vi "Normalize Elements.vi"(8 "error in (no error)":errorcluster, 9 "Hierarchies":cluster{"Hierarchy":string[]}[](array[cluster]), 10 "Elements in":refnum<class "Config Element.lvclass">[](array[class])) -> (0 "error out":errorcluster, 2 "Elements":refnum<class "Config Element.lvclass">[](array[class]))   [LabVIEW 2020, in "CDM-Config.lvlib" / "Config Manager.lvclass"]
uses:
  Config Manager.lvclass
  Config Element/Config Element.lvclass
  <vilib>/Utility/miscctls.llb/LVMapReplaceAction.ctl
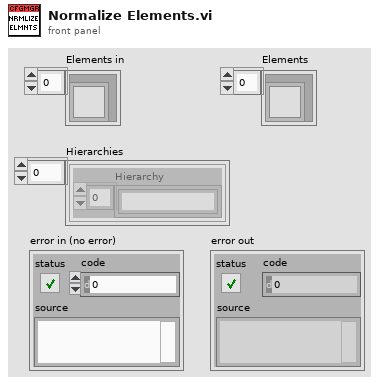
[diagram p1: front panel]
types:
  T1 = map{string[], refnum<class "Config Element.lvclass">}
  T2 = typedef "LVMapReplaceAction.ctl" = enum32{"Modify Entry only if found", "Add or Modify Entry", "Delete Entry"}
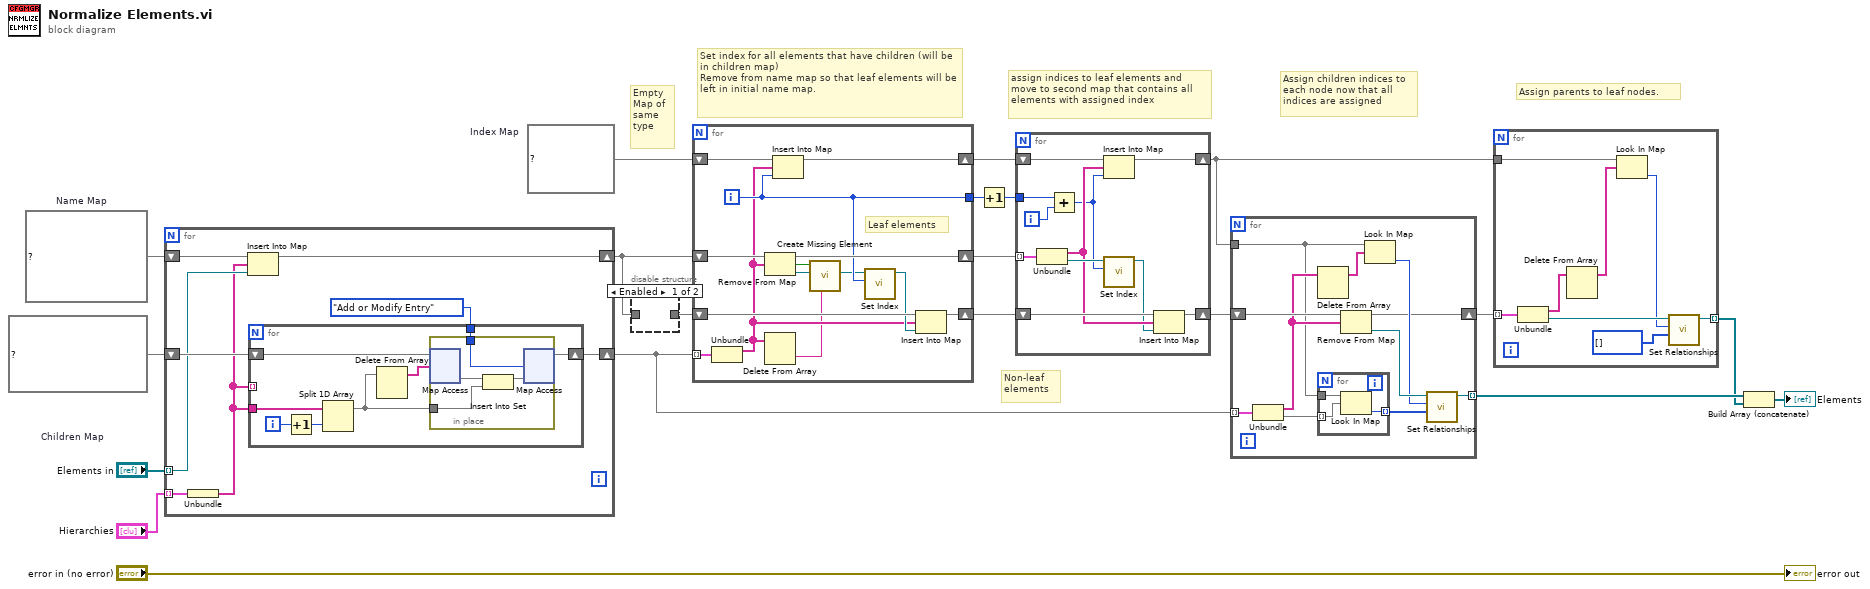
[diagram p0: block diagram]
diagram:
  w17 = map{string[], i32} {}  # Index Map
  w18 = T1 {}  # Name Map
  w19 = map{string[], set{string[]}} {}  # Children Map
  # "Assign parents to leaf nodes."
  # "Non-leaf elements"
  # "Assign children indices to each node now that all indices are assigned"
  # "assign indices to leaf elements and move to second map that contains all elements with assigned index"
  # "Set index for all elements that have children (will be in children map)\nRemove from name map so that leaf elements will be left in initial name map."
  # "Empty Map of same type"
  n1 = for {
    tunnel: "Elements in" -> [w24] mode=indexing
    shift-right: [w25] -> w11
    shift-left: w19 -> [w28]
    shift-right: [w26] -> w16
    shift-left: w18 -> [w27]
    tunnel: "Hierarchies" -> [w22] mode=indexing
    n2 = Unbundle(w22) -> ("Hierarchy"=w21:string[])
    n3 = Insert Into Map(map in=w27, key=w21, value=w24) -> (map out=w26:T1)  [unwired: 2 out]
    n4 = for {
      shift-right: [w35] -> w25
      shift-left: w28 -> [w36]
      tunnel: w21 -> [w32]
      tunnel: LVMapReplaceAction."Add or Modify Entry" ("action") -> [w29]
      tunnel: w21 -> [_] mode=indexing
      i -> [w34]
      n5 = Increment(x=w34) -> (x+1=w33:i32)
      n6 = Split 1D Array(array=w32, index=w33) -> (first subarray=w30:string[])  [unwired: 1 out]
      n7 = Delete From Array(array=w30) -> (array with subset deleted=w31:string[])  [unwired: 2 in, 1 out]
      n8 = in-place {
        in-place-border: w30 -> [w38]
        in-place-border: w29 -> [w37]
        n9 = in-place-map #1(w36, w31) -> (w40:set{string[]})  [unwired: 1 in, 1 out]
        n10 = Insert Into Set(10:w38, 11:w40) -> (3:w39:set{string[]})  [unwired: 1 out]
        n11 = in-place-map #1(w39, w37) -> (w35:map{string[], set{string[]}})  [unwired: 2 out]
      }
    }
  }
  n12 = disable-structure shown="Enabled" {
    disable-tunnel: w16 -> [_ w41]
    disable-tunnel: [_ w41] -> w15
    frame Enabled {
    }
    frame Disabled {
    }
  }
  n13 = for {
    tunnel: w11 -> [w55] mode=indexing
    shift-right: [w53] -> w14
    shift-left: w17 -> [w54]
    shift-right: [w48] -> w8
    shift-left: w16 -> [w52]
    shift-right: [w50] -> w7
    shift-left: w15 -> [w51]
    tunnel: [w47] -> w13
    i -> [w47]
    # "Leaf elements"
    n14 = Unbundle(w55) -> (w43:string[])  [unwired: 1 out]
    n15 = Remove From Map(10:w43, 11:w52) -> (1:w45:refnum<class "Config Element.lvclass">, 2:w46:bool, 3:w48:T1)
    n16 = Delete From Array(array=w43) -> (deleted portion=w42:string)  [unwired: 2 in, 1 out]
    n17 = Insert Into Map(map in=w54, key=w43, value=w47) -> (map out=w53:map{string[], i32})  [unwired: 2 out]
    n18 = call "Create Missing Element.vi"("Name"=w42, "Element in"=w45, "Create"=w46) -> ("Element"=w44:refnum<class "Config Element.lvclass">)  [unwired: 8 in]
    n19 = call "Set Index.vi"("Index"=w47, "Config Element in"=w44) -> ("Config Element out"=w49:refnum<class "Config Element.lvclass">)  [unwired: 8 in, 1 out]
    n20 = Insert Into Map(map in=w51, key=w43, value=w49) -> (map out=w50:T1)  [unwired: 2 out]
  }
  n21 = Increment(x=w13) -> (x+1=w5:i32)
  n22 = for {
    tunnel: w5 -> [w65]
    tunnel: w8 -> [w66] mode=indexing
    shift-right: [w57] -> w3
    shift-left: w14 -> [w63]
    shift-right: [w58] -> w12
    shift-left: w7 -> [w61]
    i -> [w64]
    n23 = Unbundle(w66) -> (w60:string[], "CDM-Config.lvlib:Config Element.lvclass"=w62:refnum<class "Config Element.lvclass">)
    n24 = Add(x=w65, y=w64) -> (x+y=w56:i32)
    n25 = Insert Into Map(map in=w63, key=w60, value=w56) -> (map out=w57:map{string[], i32})  [unwired: 2 out]
    n26 = call "Set Index.vi"("Index"=w56, "Config Element in"=w62) -> ("Config Element out"=w59:refnum<class "Config Element.lvclass">)  [unwired: 8 in, 1 out]
    n27 = Insert Into Map(map in=w61, key=w60, value=w59) -> (map out=w58:T1)  [unwired: 2 out]
  }
  n28 = for {
    tunnel: w3 -> [w71]
    tunnel: w11 -> [w77] mode=indexing
    tunnel: [w68] -> w10 mode=indexing
    shift-right: [w67] -> w4
    shift-left: w12 -> [w74]
    n29 = Unbundle(w77) -> (w72:string[], w76:set{string[]})
    n30 = Delete From Array(array=w72) -> (array with subset deleted=w70:string[])  [unwired: 2 in, 1 out]
    n31 = for {
      tunnel: w76 -> [w79] mode=indexing
      tunnel: w71 -> [w80]
      tunnel: [w78] -> w75 mode=indexing
      n32 = Look In Map(map=w80, key=w79) -> (value=w78:i32)  [unwired: 1 in, 1 out]
    }
    n33 = Remove From Map(10:w72, 11:w74) -> (1:w73:refnum<class "Config Element.lvclass">, 3:w67:T1)  [unwired: 1 out]
    n34 = Look In Map(map=w71, key=w70) -> (value=w69:i32)  [unwired: 1 in, 1 out]
    n35 = call "Set Relationships.vi"("Children"=w75, "Parent"=w69, "Config Element in"=w73) -> ("Config Element out"=w68:refnum<class "Config Element.lvclass">)  [unwired: 7 in, 1 out]
  }
  n36 = for {
    tunnel: w4 -> [w88] mode=indexing
    tunnel: w3 -> [w86]
    tunnel: [w84] -> w2 mode=indexing
    n37 = Unbundle(w88) -> (w87:string[], "CDM-Config.lvlib:Config Element.lvclass"=w85:refnum<class "Config Element.lvclass">)
    n38 = Delete From Array(array=w87) -> (array with subset deleted=w83:string[])  [unwired: 2 in, 1 out]
    n39 = Look In Map(map=w86, key=w83) -> (value=w82:i32)  [unwired: 1 in, 1 out]
    n40 = call "Set Relationships.vi"("Children"=i32[] [], "Parent"=w82, "Config Element in"=w85) -> ("Config Element out"=w84:refnum<class "Config Element.lvclass">)  [unwired: 7 in, 1 out]
  }
  n41 = Build Array (concatenate)(w10, w2) -> (→"Elements":refnum<class "Config Element.lvclass">[])
  "error out" <- "error in (no error)"
